vi "Read Response.vi"(8 "error in (no error)":errorcluster, 11 "VISA resource name":refnum<visa-resource-name>) -> (0 "error out":errorcluster, 2 "Confirmation Response":string, 3 "VISA resource name out":refnum<visa-resource-name>)   [LabVIEW 2024, in "Micron Optics sm130.lvlib"]
doc: "Reads the response from the instrument. Error responses will be passes through the error cluster. Confirmation response string output is for convinience and can be ignored."
uses:
  Micron Optics sm130.lvlib
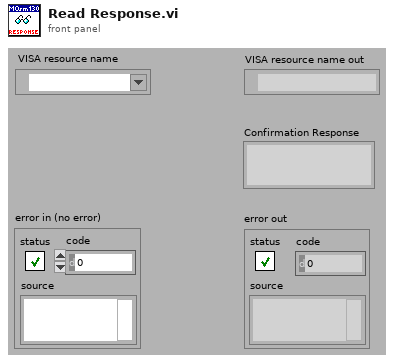
[diagram p1: front panel]
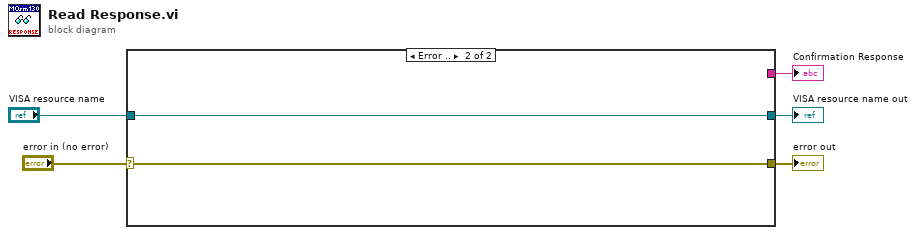
[diagram p0: block diagram]
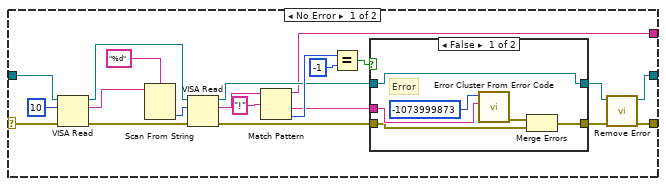
[diagram p2: hidden frame]
diagram:
  n1 = case shown="Error .." "error in (no error)" {
    selector: "error in (no error)" -> [w6 w35]
    tunnel: "VISA resource name" -> [w24 w36]
    tunnel: [w11 _] -> w4
    tunnel: [w9 w35] -> w3
    tunnel: [w8 w36] -> w2
    frame No Error {
      n2 = VISA Read(VISA resource name=w24, byte count=u32 10, error in (no error)=w6) -> (VISA resource name out=w25:refnum<visa-resource-name>, read buffer=w22:string, error out=w26:errorcluster)  [unwired: 1 out]
      n3 = Scan From String(format string="%d", input string=w22) -> (output 1=w21:i32)  [unwired: 3 in, 3 out]
      n4 = VISA Read(VISA resource name=w25, byte count=w21, error in (no error)=w26) -> (VISA resource name out=w13:refnum<visa-resource-name>, read buffer=w20:string, error out=w14:errorcluster)  [unwired: 1 out]
      n5 = Match Pattern(string=w20, regular expression="!") -> (before substring=w11:string, after substring=w15:string, offset past match=w18:i32)  [unwired: 1 in, 1 out]
      n6 = Equal?(x=w18, y=-1) -> (x = y?=w16:bool)
      n7 = case shown="False" w16 {
        tunnel: w15 -> [w31 _]
        tunnel: w14 -> [w29 w33]
        tunnel: w13 -> [w28 w34]
        tunnel: [w28 w34] -> w7
        tunnel: [w27 w33] -> w10
        frame False {
          # "Error"
          n8 = call <vilib>:"Error Cluster From Error Code.vi"("error message (\"\")"=w31, "error code (0)"=-1073999873) -> ("error out"=w30:errorcluster)  [unwired: 7 in]
          n9 = Merge Errors(w30, w29) -> (w27:errorcluster)
        }
        frame True {
          # "No Error"
        }
      }
      n10 = call "Remove Error.vi"("error in (no error)"=w10, "VISA resource name"=w7) -> ("error out"=w9:errorcluster, "VISA resource name out"=w8:refnum<visa-resource-name>)  [unwired: 8 in]
    }
    frame Error {
    }
  }
  "VISA resource name out" <- w2
  "error out" <- w3
  "Confirmation Response" <- w4
